vi "Radwag Commands Definition.vi"() -> ()   [LabVIEW 2016]
panel:
  in  "name & pwd":string
  in  "Value":i8
  out "String":string
  in  "cmd":T1(ring)=enum."AutoZero"
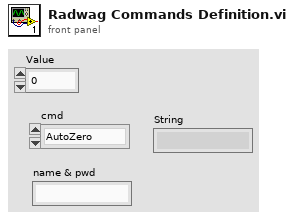
[diagram p1: front panel]
types:
  T1 = enum16{"nop", "Tare", "Zero", "Lock", "Unlock", "AutoZero", "SetFilter", "Login", "Logout"}
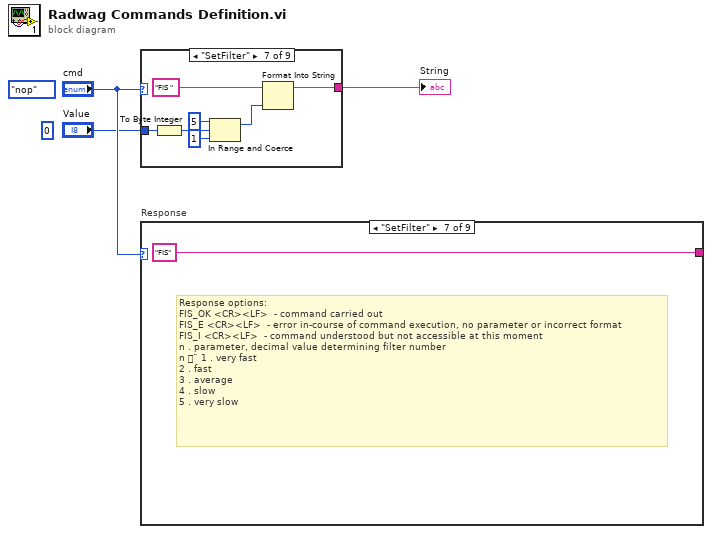
[diagram p0: block diagram]
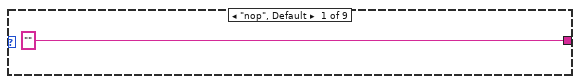
[diagram p2: hidden frame]
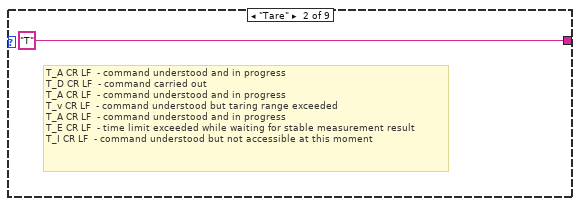
[diagram p3: hidden frame]
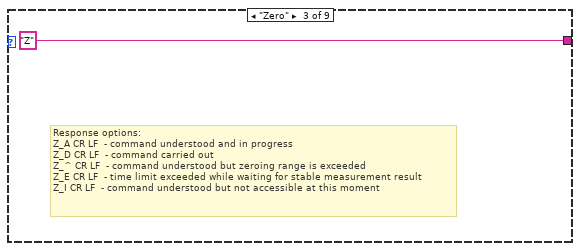
[diagram p4: hidden frame]
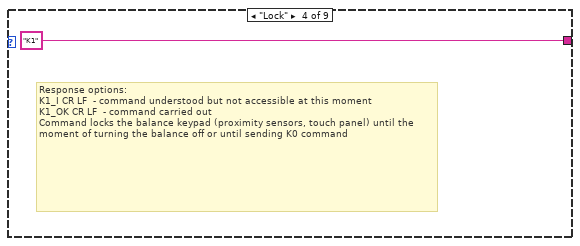
[diagram p5: hidden frame]
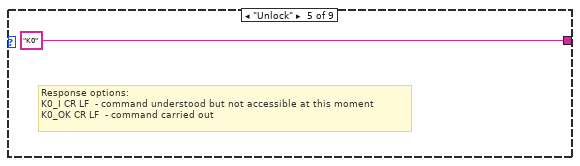
[diagram p6: hidden frame]
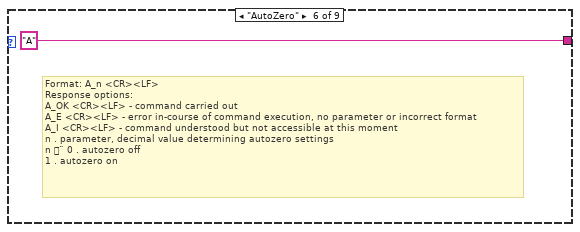
[diagram p7: hidden frame]
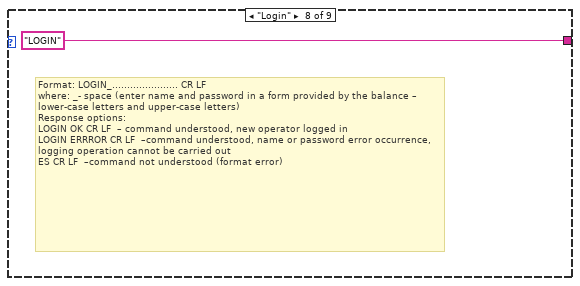
[diagram p8: hidden frame]
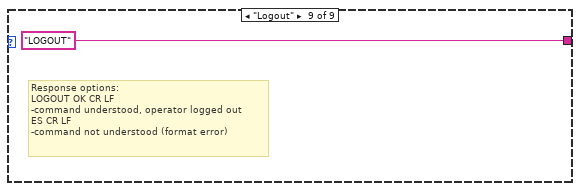
[diagram p9: hidden frame]
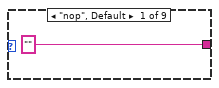
[diagram p10: hidden frame]
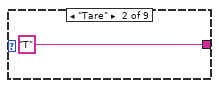
[diagram p11: hidden frame]
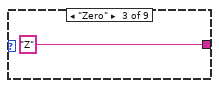
[diagram p12: hidden frame]
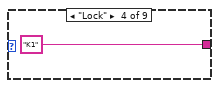
[diagram p13: hidden frame]
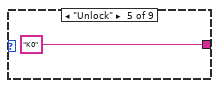
[diagram p14: hidden frame]
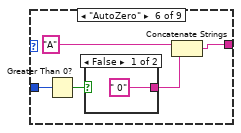
[diagram p15: hidden frame]
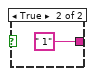
[diagram p16: hidden frame]
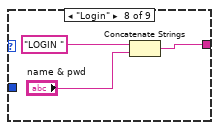
[diagram p17: hidden frame]
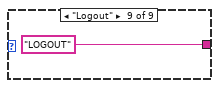
[diagram p18: hidden frame]
diagram:
  (unwired) i8 0 ("Value")
  (unwired) T1."nop" ("cmd")
  n1 = case shown="\"SetFilter\"" "cmd" {
    tunnel: ["" "T" "Z" "K1" "K0" w10 w21 w24 "LOGOUT"] -> w3
    tunnel: "Value" -> [_ _ _ _ _ w13 w20 _ _]
    frame "nop", Default {
    }
    frame "Tare" {
    }
    frame "Zero" {
    }
    frame "Lock" {
    }
    frame "Unlock" {
    }
    frame "AutoZero" {
      n2 = Greater Than 0?(x=w13) -> (x > 0?=w12:bool)
      n3 = case shown="False" w12 {
        tunnel: [" 0" " 1"] -> w9
        frame False {
        }
        frame True {
        }
      }
      n4 = Concatenate Strings("A", w9) -> (w10:string)
    }
    frame "SetFilter" {
      n5 = To Byte Integer(number=w20) -> (8bit integer=w19:i8)
      n6 = In Range and Coerce(upper limit=i8 5, x=w19, lower limit=i8 1) -> (coerced(x)=w18:i8)  [unwired: 1 out]
      n7 = Format Into String(initial string="FIS ", w18) -> (resulting string=w21:string)  [unwired: 2 in, 1 out]
    }
    frame "Login" {
      n8 = Concatenate Strings("LOGIN ", "name & pwd") -> (w24:string)
    }
    frame "Logout" {
    }
  }
  "String" <- w3
  n9 = case "Response" shown="\"SetFilter\"" "cmd" {
    tunnel: ["" "T" "Z" "K1" "K0" "A" "FIS" "LOGIN" "LOGOUT"] -> _
    frame "nop", Default {
    }
    frame "Tare" {
      # "T_A CR LF  - command understood and in progress\nT_D CR LF  - command carried out\nT_A CR LF  - command understood and in progress\nT_v CR LF  - command understood but taring range exceeded\nT_A CR LF  - command understood and in progress\nT_E CR LF  - time limit exceeded while waiting for stable measurement result\nT_I CR LF  - command understood but not accessible at this moment"
    }
    frame "Zero" {
      # "Response options:\nZ_A CR LF  - command understood and in progress\nZ_D CR LF  - command carried out\nZ_^ CR LF  - command understood but zeroing range is exceeded\nZ_E CR LF  - time limit exceeded while waiting for stable measurement result\nZ_I CR LF  - command understood but not accessible at this moment"
    }
    frame "Lock" {
      # "Response options:\nK1_I CR LF  - command understood but not accessible at this moment\nK1_OK CR LF  - command carried out\nCommand locks the balance keypad (proximity sensors, touch panel) until the moment of turning the balance off or until sending K0 command"
    }
    frame "Unlock" {
      # "Response options:\nK0_I CR LF  - command understood but not accessible at this moment\nK0_OK CR LF  - command carried out"
    }
    frame "AutoZero" {
      # "Format: A_n <CR><LF>\nResponse options:\nA_OK <CR><LF> - command carried out\nA_E <CR><LF> - error in-course of command execution, no parameter or incorrect format\nA_I <CR><LF> - command understood but not accessible at this moment\nn . parameter, decimal value determining autozero settings\nn ¨ 0 . autozero off\n1 . autozero on"
    }
    frame "SetFilter" {
      # "Response options:\nFIS_OK <CR><LF>  - command carried out\nFIS_E <CR><LF>  - error in-course of command execution, no parameter or incorrect format\nFIS_I <CR><LF>  - command understood but not accessible at this moment\nn . parameter, decimal value determining filter number\nn ¨ 1 . very fast\n2 . fast\n3 . average\n4 . slow\n5 . very slow"
    }
    frame "Login" {
      # "Format: LOGIN_...................... CR LF\nwhere: _- space (enter name and password in a form provided by the balance – lower-case letters and upper-case letters)\nResponse options:\nLOGIN OK CR LF  – command understood, new operator logged in\nLOGIN ERRROR CR LF  –command understood, name or password error occurrence, logging operation cannot be carried out\nES CR LF  –command not understood (format error)"
    }
    frame "Logout" {
      # "Response options:\nLOGOUT OK CR LF\n-command understood, operator logged out\nES CR LF\n-command not understood (format error)"
    }
  }
